vi "2fer.vi"() -> ()   [LabVIEW 2014]
uses:
  Sensors/Adafruit INA219/INA219 Measurements.ctl
  <vilib>/myRIO/Instrument Drivers/Onboard IO/DIO/typedefs/DIO Reference.ctl
  <vilib>/myRIO/Common/Instrument Driver Framework/Utilities/typedefs/myRIO Generic Hardware Reference.ctl
  <vilib>/myRIO/Common/Instrument Driver Framework/Utilities/typedefs/Hardware Version Enum.ctl
  <vilib>/myRIO/Common/Instrument Driver Framework/Utilities/typedefs/myRIO v1.0 Reference.ctl
  <vilib>/myRIO/Common/Instrument Driver Framework/Utilities/typedefs/Generic FPGA Reference.ctl
  <vilib>/myRIO/Common/Instrument Driver Framework/myRIO v1.0/DIO/typedefs/DIO Channels List.ctl
  <vilib>/myRIO/Common/Instrument Driver Framework/myRIO v1.0/DIO/typedefs/DIO Channels Enum.ctl
  <vilib>/userdefined/High Color/nirio_resource_hc.ctl
  <vilib>/myRIO/Common/Instrument Driver Framework/Utilities/vis/Is FPGA Ref Available.vi
  <vilib>/myRIO/Common/Instrument Driver Framework/myRIO v1.0/DIO/vis/myRIO v1.1 Open DIO.vi
  <vilib>/myRIO/Instrument Drivers/Onboard IO/DIO/vis/Write.vi
  <vilib>/myRIO/Common/Instrument Driver Framework/Utilities/vis/Validate Channels.vi
  <vilib>/myRIO/Common/Instrument Driver Framework/myRIO v1.0/DIO/vis/myRIO v1.0 Reserve DIO.vi
  <vilib>/myRIO/Common/Instrument Driver Framework/myRIO v1.0/Resource Manager/vis/myRIO v1.0 Reserve Channel List.vi
  <vilib>/myRIO/Common/Instrument Driver Framework/myRIO v1.0/DIO/vis/myRIO v1.0 Build MUX Configuration DIO.vi
  <vilib>/myRIO/Common/Instrument Driver Framework/myRIO v1.0/Resource Manager/vis/myRIO v1.0 Reserve Channel.vi
  <vilib>/myRIO/Common/Instrument Driver Framework/myRIO v1.0/Resource Manager/vis/myRIO v1.0 Unreserve Channel.vi
  <vilib>/myRIO/Common/Instrument Driver Framework/myRIO v1.0/Resource Manager/vis/myRIO v1.0 Create Configuration List.vi
  <vilib>/myRIO/Common/Instrument Driver Framework/myRIO v1.0/Resource Manager/vis/myRIO v1.0 Build Mutex Name.vi
  <vilib>/Utility/VariantDataType/GetNumericInfo.vi
  <vilib>/Utility/error.llb/Error Cluster From Error Code.vi
  <vilib>/myRIO/Common/Instrument Driver Framework/myRIO v1.0/myRIO v1.1 Open.vi
  <vilib>/myRIO/Common/Instrument Driver Framework/Utilities/vis/IO Manager.vi
  <vilib>/myRIO/Common/Instrument Driver Framework/Utilities/vis/Configuration Manager.vi
  <vilib>/myRIO/Common/Instrument Driver Framework/myRIO v1.0/Resource Manager/vis/myRIO v1.0 Configure IO.vi
  <vilib>/myRIO/Common/Instrument Driver Framework/myRIO v1.0/myRIO v1.0 Close.vi
  <vilib>/myRIO/Common/Instrument Driver Framework/myRIO v1.0/DIO/vis/myRIO v1.0 Write DIO.vi
  <vilib>/MakerHub/LINX/Public/Utilities/Open Local.vi
  <vilib>/myRIO/Express VI/Onboard IO/DO/DO Express VI.xnode
  <vilib>/myRIO/Instrument Drivers/Onboard IO/DIO/vis/myRIO DIO Open.xnode
  <vilib>/MakerHub/LINX/LMH-LINX.lvlib
  <vilib>/myRIO/Instrument Drivers/Onboard IO/DIO/DIO.lvlib
panel:
  out "Pressure":i32(graph)
  out "Thermometer":dbl(slide) scale=0.0..100.0
  in  "I2C Slave Address 2":u8=119 format="%x"
  in  "I2C Slave Address":u8=64 format="%x"
  out "V & P Monitor":cluster{"Voltage (Total)":dbl, "Power":dbl}(graph)
  out "Measurements":T1 {"Current" format="%#.3g A"; "Power" format="%#.3g W"; "Shunt Voltage" format=" %#.3g V"; "Bus Voltage" format="%#.3g V"; "Voltage (Total)" format="%#.3g V"}
  in  "I2C Channel":u8=1
  out "Error Out":errorcluster
  out "ToF Loop Rate":u32
  in  "Wait (ms)":u32=10
  in  "Stop":bool
  # "INA219"
  # "BMP180"
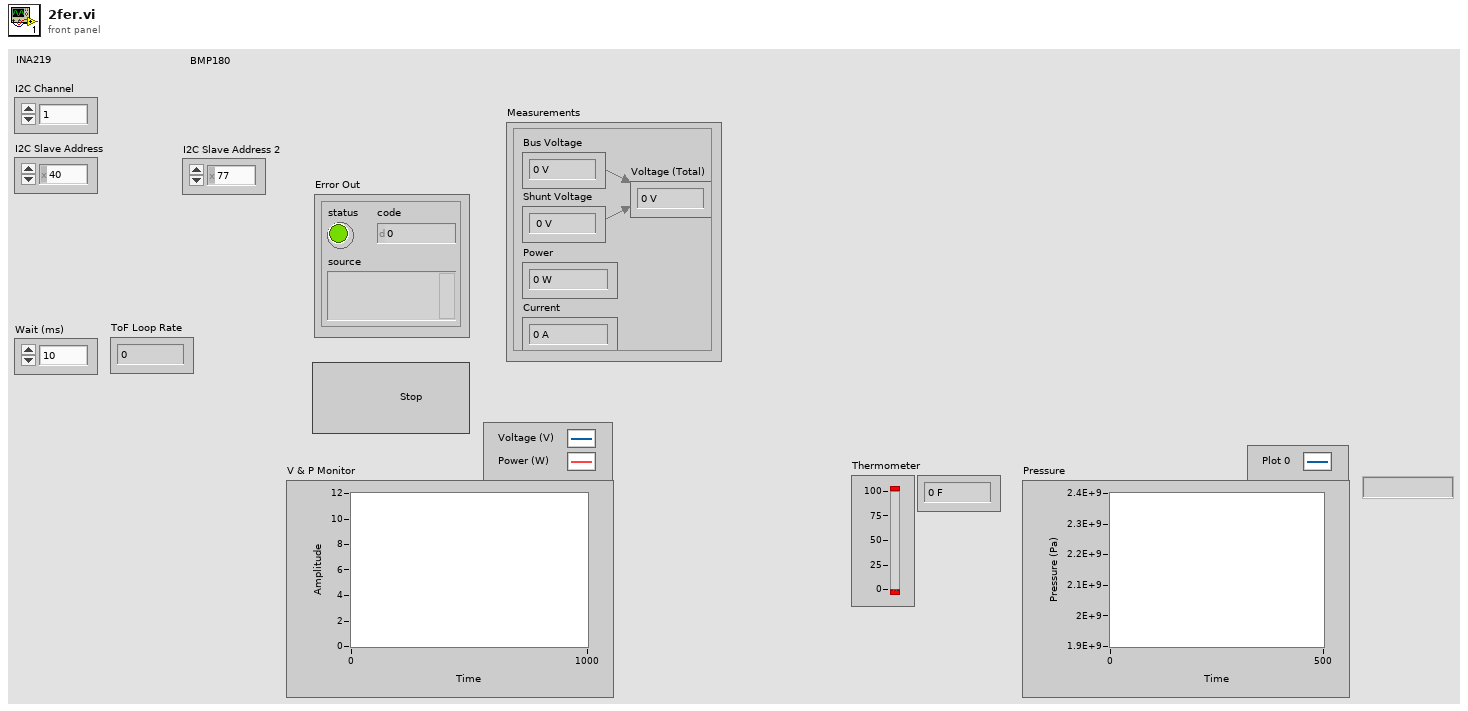
[diagram p1: front panel]
types:
  T1 = typedef "INA219 Measurements.ctl" = cluster{"Voltage (Total)":dbl, "Bus Voltage":dbl, "Shunt Voltage":dbl, "Power":dbl, "Current":dbl}
  T2 = typedef "LMH-LINX.lvlib/LINX Ref.ctl" = cluster{"IO":T3, "Interface":T4, "LINX Device Config":T5}
  T3 = typedef "LMH-LINX.lvlib/Platform.ctl" = enum16{"Remote", "Local"}
  T4 = typedef "LMH-LINX.lvlib/Interface.ctl" = enum16{"Serial", "TCP"}
  T5 = typedef "LMH-LINX.lvlib/Device.lvlib/LINX Device Config.ctl" = cluster{"Interface":T4, "COM Port":refnum<visa-resource-name>, "TCP Configuration":T6, "Device Family":u8, "Device ID":u8, "Device Name":string, "TCP Ref":refnum<k5>, "Channels":T7}
  T6 = typedef "LMH-LINX.lvlib/Device.lvlib/TCP Config.ctl" = cluster{"IP Address":string, "Port":u16}
  T7 = typedef "LMH-LINX.lvlib/Channels.ctl" = cluster{"DI":u8[], "DO":u8[], "AI":u8[], "AO":u8[], "PWM":u8[], "QE":u8[], "UART":u8[], "I2C 2":u8[], "SPI":u8[], "CAN":u8[], "Servo":u8[], "AI Ref (V)":dbl, "AI Resolution (Bits)":u8, "AO Ref (V)":dbl, "AO Resolution (Bits)":u8}
  T8 = typedef "INA219 Config Options.ctl" = cluster{"Reset bit":u8, "Bus Voltage Range":u8, "PGA/Shunt Voltage Gain":u8, "Bus Voltage ADC Settings":u8, "Shunt Voltage ADC Settings":u8, "Mode":u8, "Calibration Value":u16}
  T9 = typedef "BMP180 Config Options.ctl" = cluster{"Mode":enum8{"Ultra Low Power", "Standard", "High Resolution", "Ultra High Resolution"}, "Cal Coefs":cluster{"AC1":cluster{"Addr:":u8, "Val:":u16}, "AC2":cluster{"Addr:":u8, "Val:":u16}, "AC3":cluster{"Addr:":u8, "Val:":u16}, "AC4":cluster{"Addr:":u8, "Val:":u16}, "AC5":cluster{"Addr:":u8, "Val:":u16}, "AC6":cluster{"Addr:":u8, "Val:":u16}, "B1":cluster{"Addr:":u8, "Val:":u16}, "B2":cluster{"Addr:":u8, "Val:":u16}, "MB":cluster{"Addr:":u8, "Val:":u16}, "MC":cluster{"Addr:":u8, "Val:":u16}, "MD":cluster{"Addr:":u8, "Val:":u16}}}
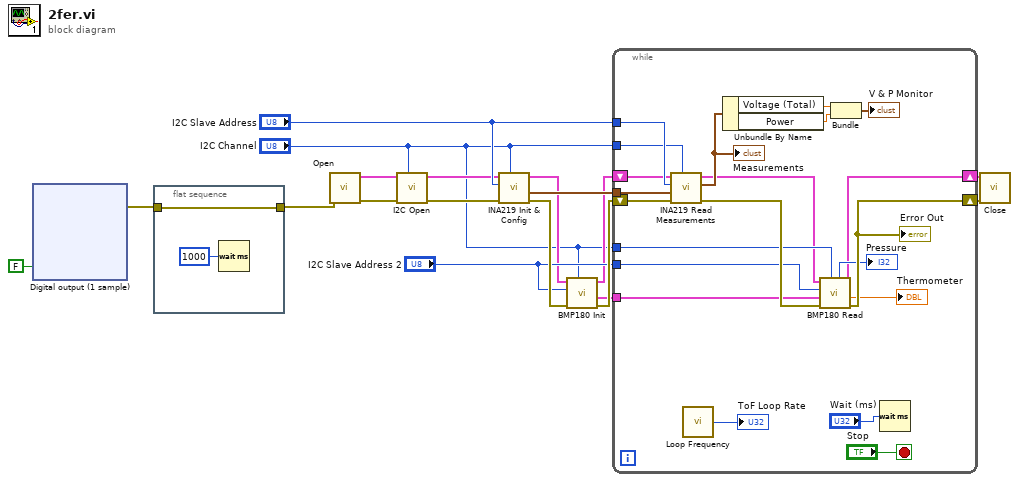
[diagram p0: block diagram]
diagram:
  n1 = xnode "Digital output (1 sample)"("Sensor Power (B/DIO7 (Pin 25))"=FALSE) -> ("error out"=w13:errorcluster)  [unwired: 1 in]
  n2 = flat-sequence {
    tunnel: w13 -> [w20]
    tunnel: [w20] -> w12
    frame #0 {
      n3 = Wait (ms)(milliseconds to wait=u32 1000) -> ()  [unwired: 1 out]
    }
  }
  n4 = call-poly <vilib>:"Open.vi"("Error In"=w12) -> ("Error Out"=w17:errorcluster, "LINX Resource"=w18:T2)  [unwired: 8 in, 1 out]
  n5 = call <vilib>:"I2C Open.vi"("I2C Channel (0)"="I2C Channel", "Error In"=w17, "LINX Resource"=w18) -> ("Error Out"=w2:errorcluster, "LINX Resource"=w3:T2)  [unwired: 7 in]
  n6 = call "INA219 Init & Config.vi"("I2C Channel"="I2C Channel", "error in (no error)"=w2, "I2C Slave Address"="I2C Slave Address", "LINX Resource in"=w3) -> ("error out"=w10:errorcluster, "INA219 Config Options"=w11:T8, "LINX Resource out"=w6:T2)  [unwired: 5 in]
  n7 = call "BMP180 Init.vi"("I2C Channel"="I2C Channel", "error in (no error)"=w10, "I2C Slave Address"="I2C Slave Address 2", "LINX Resource in"=w6) -> ("error out"=w9:errorcluster, "BMP180 Config Options"=w7:T9, "LINX Resource out"=w5:T2)  [unwired: 5 in]
  n8 = while {
    shift-right: [w21] -> w16
    shift-left: w5 -> [w36]
    shift-right: [w29] -> w15
    shift-left: w9 -> [w35]
    tunnel: "I2C Channel" -> [w38]
    tunnel: "I2C Slave Address" -> [w39]
    tunnel: w11 -> [w37]
    tunnel: "I2C Channel" -> [w27]
    tunnel: "I2C Slave Address 2" -> [w26]
    tunnel: w7 -> [w25]
    stop <- "Stop" stop-if-true
    n9 = call "INA219 Read Measurements.vi"("I2C Channel"=w38, "error in (no error)"=w35, "INA219 Config Options"=w37, "I2C Slave Address"=w39, "LINX Resource in"=w36) -> ("error out"=w28:errorcluster, "Measurements"=w34:T1, "LINX Resource"=w22:T2)  [unwired: 4 in]
    "Measurements" <- w34
    n10 = call <vilib>:"Loop Frequency.vi"() -> ("Loop Rate (Hz)"=→"ToF Loop Rate":u32)
    n11 = Unbundle By Name(w34) -> ("Voltage (Total)"=w32:dbl, "Power"=w31:dbl)
    n12 = call "BMP180 Read.vi"("I2C Channel"=w27, "error in (no error)"=w28, "BMP180 Config"=w25, "I2C Slave Address"=w26, "LINX Resource in"=w22) -> ("error out"=w29:errorcluster, "Temperature (F)"=→"Thermometer":dbl, "LINX Resource"=w21:T2, "Pressure"=→"Pressure":i32)  [unwired: 2 in, 1 out]
    "Error Out" <- w29
    n13 = Bundle("Voltage (Total)"=w32, "Power"=w31) -> (→"V & P Monitor":cluster{"Voltage (Total)":dbl, "Power":dbl})  [unwired: 1 in]
    n14 = Wait (ms)(milliseconds to wait="Wait (ms)") -> ()  [unwired: 1 out]
  }
  n15 = call <vilib>:"Close.vi"("Error In"=w15, "LINX Resource"=w16) -> ()  [unwired: 9 in, 1 out]
